vi "polhemus graph.vi"() -> ()   [LabVIEW 2018]
panel:
  out "XY Graph":cluster{dbl, "x":sgl}[](graph)
  in  "XYZAER":T1(array[cluster]) {"r" format="%1_6f"; "e" format="%1_6f"; "a" format="%1_6f"; "z" format="%1_6f"; "y" format="%1_6f"; "x" format="%1_6f"}
  out "Connected":bool
  out "Start Time Text":string
  out "Stop Time Text":string
  out "Elapsed Time Text":string
  out "HostFrameCount":u32
  out "Running":bool
  out "Loop Iter":i32
  out "PnoData":bool
  in  "stop":bool
  out "error out":errorcluster {"code" format="%.0x"}
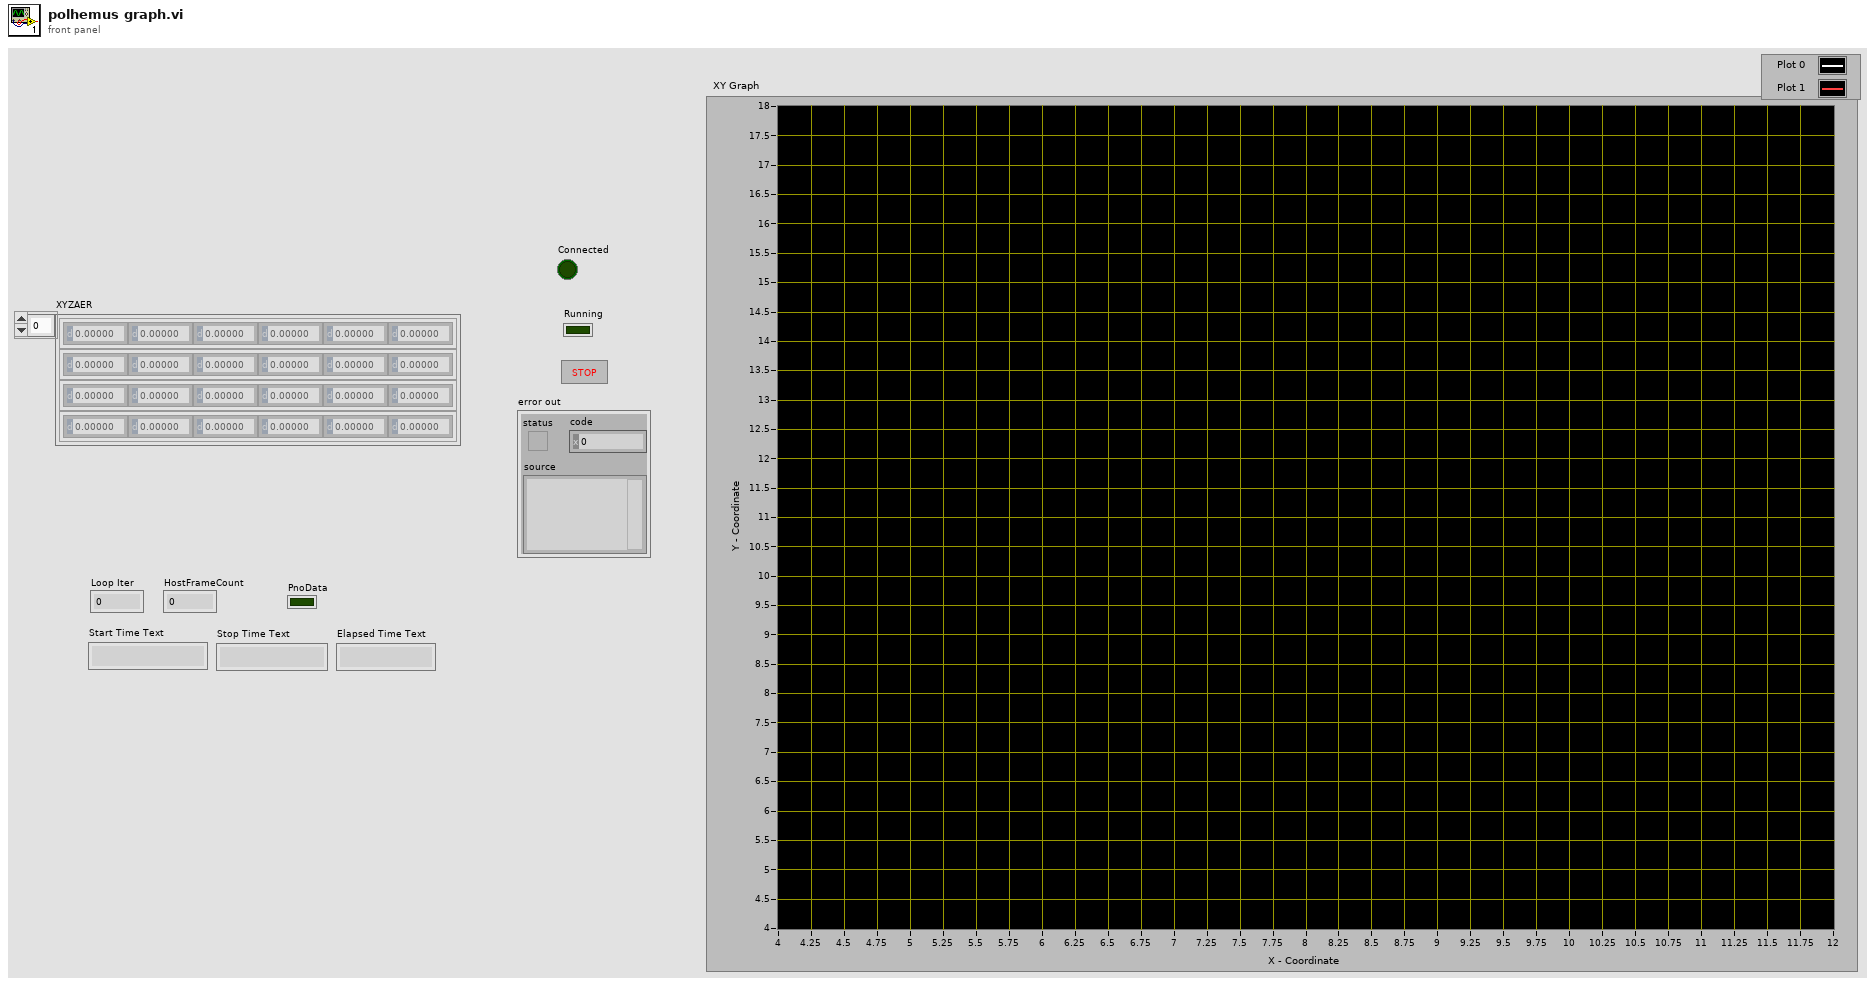
[diagram p1: front panel]
types:
  T1 = cluster{"x":sgl, "y":sgl, "z":sgl, "a":sgl, "e":sgl, "r":sgl}[]
  T2 = cluster{"x":sgl, "y":sgl, "z":sgl, "a":sgl, "e":sgl, "r":sgl}
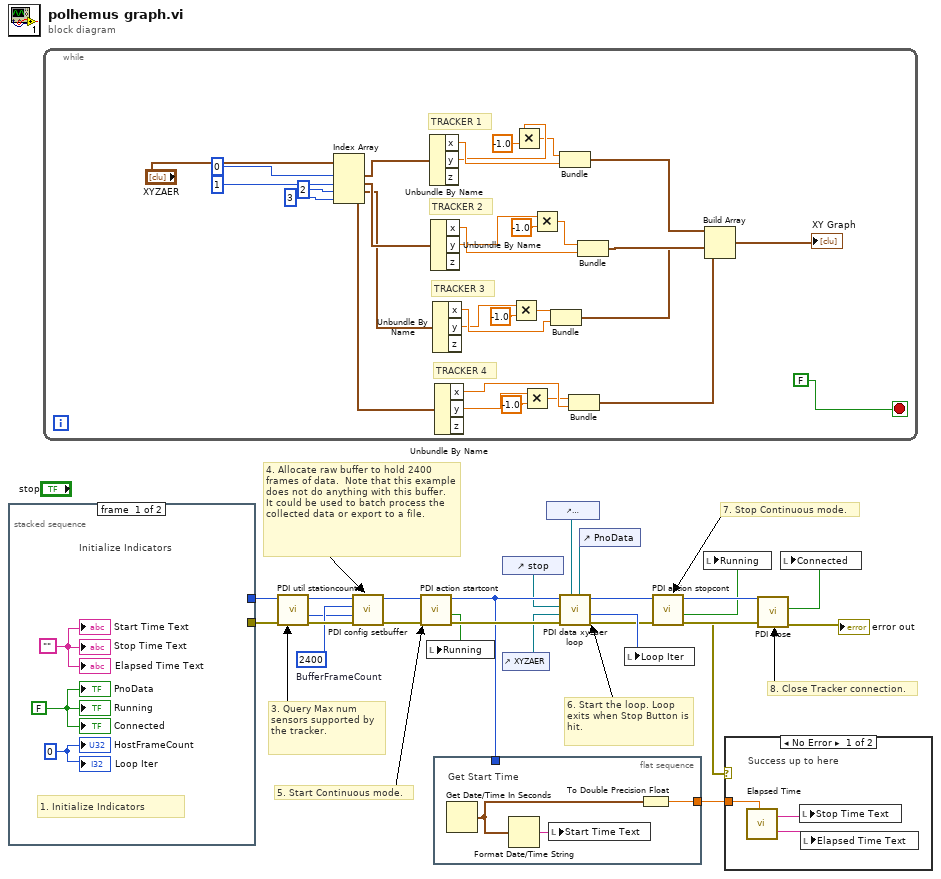
[diagram p0: block diagram]
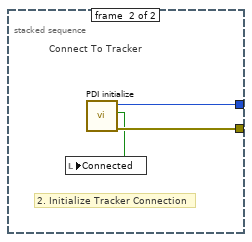
[diagram p3: hidden frame]
diagram:
  w3 = 2400  # BufferFrameCount
  # "8. Close Tracker connection."
  # "3. Query Max num sensors supported by the tracker."
  # "4. Allocate raw buffer to hold 2400 frames of data.  Note that this example does not do anything with this buffer.  It could be used to batch process the collected data or export to a file."
  # "5. Start Continuous mode."
  # "7. Stop Continuous mode."
  # "6. Start the loop. Loop exits when Stop Button is hit."
  n1 = stacked-sequence {
    tunnel: [_ w30] -> w7
    tunnel: [_ w29] -> w6
    frame #0 {
      w25 = 0
      w26 = FALSE
      w27 = ""
      # "Initialize Indicators"
      # "1. Initialize Indicators"
      "Connected" <- w26
      "Start Time Text" <- w27
      "Stop Time Text" <- w27
      "Elapsed Time Text" <- w27
      "HostFrameCount" <- w25
      "Running" <- w26
      "Loop Iter" <- w25
      "PnoData" <- w26
    }
    frame #1 {
      # "Connect To Tracker"
      # "2. Initialize Tracker Connection"
      n2 = call <instrlib>:"PDI initialize.vi"() -> ("error out"=w29:errorcluster, "Connected"=w28:bool, "pDev"=w30:u32)  [unwired: 1 in, 4 out]
      n3 = local write "Connected"(w28) -> ()
    }
  }
  n4 = while {
    stop <- FALSE stop-if-true
    # "TRACKER 4"
    # "TRACKER 3"
    # "TRACKER 2"
    # "TRACKER 1"
    n5 = Index Array(array="XYZAER", index #1=0 ("index"), index #2=1 ("index"), index #3=2 ("index"), index #4=3 ("index")) -> (element #1=w55:T2, element #2=w54:T2, element #3=w53:T2, element #4=w52:T2)
    n6 = Unbundle By Name(w55) -> ("x"=w42:sgl, "y"=w41:sgl)  [unwired: 1 out]
    n7 = Unbundle By Name(w54) -> ("x"=w39:sgl, "y"=w38:sgl)  [unwired: 1 out]
    n8 = Unbundle By Name(w53) -> ("x"=w36:sgl, "y"=w35:sgl)  [unwired: 1 out]
    n9 = Unbundle By Name(w52) -> ("x"=w33:sgl, "y"=w32:sgl)  [unwired: 1 out]
    n10 = Multiply(x=w35, y=-1.0) -> (x*y=w34:dbl)
    n11 = Multiply(x=w41, y=sgl -1.0) -> (x*y=w40:sgl)
    n12 = Multiply(x=w32, y=-1.0) -> (x*y=w31:dbl)
    n13 = Multiply(x=w38, y=-1.0) -> (x*y=w37:dbl)
    n14 = Bundle(w34, "x"=w36) -> (w49:cluster{dbl, "x":sgl})  [unwired: 1 in]
    n15 = Bundle(w40, "x"=w42) -> (w51:cluster{sgl, "x":sgl})  [unwired: 1 in]
    n16 = Bundle(w31, "x"=w33) -> (w48:cluster{dbl, "x":sgl})  [unwired: 1 in]
    n17 = Bundle(w37, "x"=w39) -> (w50:cluster{dbl, "x":sgl})  [unwired: 1 in]
    n18 = Build Array(w51, w50, w49, w48) -> (→"XY Graph":cluster{dbl, "x":sgl}[])
  }
  n19 = call <instrlib>:"PDI util stationcount.vi"("error in (no error)"=w6, "pDev"=w7) -> ("error out"=w5:errorcluster, "dup pDev"=w4:u32, "MaxCount"=w2:i32)  [unwired: 7 out]
  n20 = call <instrlib>:"PDI config setbuffer.vi"("error in (no error)"=w5, "Max sensors"=w2, "FrameCount"=w3, "pDev"=w4) -> ("error out"=w14:errorcluster, "dup pDev"=w15:u32)  [unwired: 6 out]
  n21 = call <instrlib>:"PDI action startcont.vi"("error in (no error)"=w14, "pDev"=w15) -> ("error out"=w21:errorcluster, "Running"=w13:bool, "dup pDev"=w20:u32)  [unwired: 7 out]
  n22 = local write "Running"(w13) -> ()
  n23 = flat-sequence {
    tunnel: w20 -> [_]
    tunnel: [w62] -> w16
    frame #0 {
      # "Get Start Time"
      n24 = Get Date/Time In Seconds() -> (seconds since 1Jan1904=w63:timestamp)
      n25 = Format Date/Time String(seconds (now)=w63) -> (date/time string=w64:string)  [unwired: 2 out]
      n26 = local write "Start Time Text"(w64) -> ()
      n27 = To Double Precision Float(number=w63) -> (double precision float=w62:dbl)
    }
  }
  n28 = control-ref of="stop"() -> (w19:refnum<vi>)
  n29 = control-ref of="XYZAER"() -> (w10:refnum<vi>)
  n30 = control-ref of="HostFrameCount"() -> (w11:refnum<vi>)
  n31 = control-ref of="PnoData"() -> (w1:refnum<vi>)
  n32 = call <instrlib>:"PDI data xyzaer loop.vi"("Data Ready Refnum"=w1, "FrameCount Ctl Ref"=w11, "error in (no error)"=w21, "xyzaer array\nRefnum"=w10, "Stop Ctl Ref"=w19, "pDev"=w20) -> ("error out"=w8:errorcluster, "Loop Iter"=w12:i32, "dup pDev"=w9:u32)  [unwired: 3 out]
  n33 = local write "Loop Iter"(w12) -> ()
  n34 = call <instrlib>:"PDI action stopcont.vi"("error in (no error)"=w8, "pDev"=w9) -> ("error out"=w17:errorcluster, "Running"=w22:bool, "dup pDev"=w23:u32)  [unwired: 7 out]
  n35 = local write "Running"(w22) -> ()
  n36 = case shown="No Error" w8 {
    tunnel: w16 -> [w65 _]
    frame No Error {
      # "Success up to here"
      n37 = call "Elapsed Time"("Set Start Time (s)"=w65) -> ("Present Text"=w67:string, "Elapsed Time Text"=w66:string)  [unwired: 4 in, 13 out]
      n38 = local write "Stop Time Text"(w67) -> ()
      n39 = local write "Elapsed Time Text"(w66) -> ()
    }
    frame Error {
      # "Error somewhere;\nStop Time is irrelevant"
    }
  }
  n40 = call <instrlib>:"PDI close.vi"("error in (no error)"=w17, "pDev"=w23) -> ("error out"=→"error out":errorcluster, "connected"=w18:bool)  [unwired: 8 out]
  n41 = local write "Connected"(w18) -> ()
